vi "Set LV Color.vi"(8 "error in (no error)":errorcluster, 10 "Color (black)":u32(colorbox), 11 "RGB Color.lvclass in":refnum<class "RGB Color.lvclass">) -> (0 "error out":errorcluster, 3 "RGB Color.lvclass out":refnum<class "RGB Color.lvclass">)   [LabVIEW 2018, in "RGB Color.lvclass"]
doc: "A method to set the color from a LabVIEW color value. If the same color cannot be shown in the color model, the closest color will be selected."
uses:
  RGB Color.lvclass
  RGB Color.lvclass/RGB Color.ctl
panel:
  # "expressionflow.com"
  # "Copyright (c) 2008 Tomi Maila. All rights reserved."
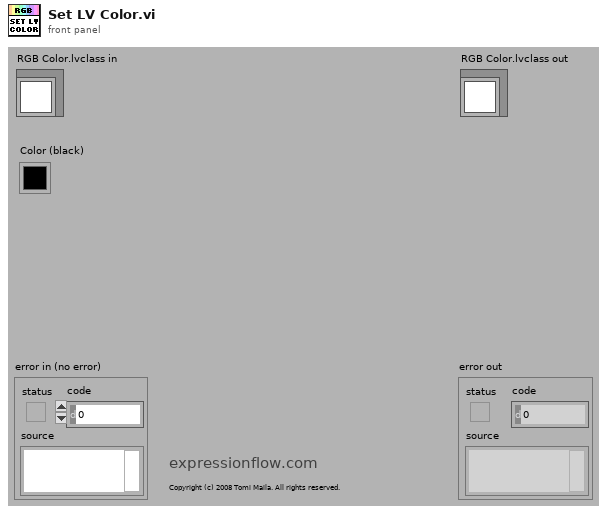
[diagram p1: front panel]
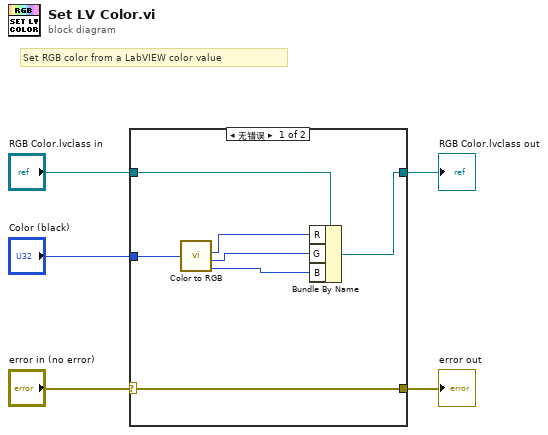
[diagram p0: block diagram]
diagram:
  # "Set RGB color from a LabVIEW color value"
  n1 = case shown="无错误" "error in (no error)" {
    selector: "error in (no error)" -> [w12 w13]
    tunnel: [w12 w13] -> w4
    tunnel: "RGB Color.lvclass in" -> [w11 w14]
    tunnel: [w10 w14] -> w2
    tunnel: "Color (black)" -> [w9 _]
    frame No Error {
      n2 = call <vilib>:"Color to RGB.vi"("Color"=w9) -> ("R"=w8:u8, "G"=w7:u8, "B"=w6:u8)  [unwired: 1 out]
      n3 = Bundle By Name(cluster=w11, "R"=w8, "G"=w7, "B"=w6) -> (w10:refnum<class "RGB Color.lvclass">)
    }
    frame Error {
    }
  }
  "error out" <- w4
  "RGB Color.lvclass out" <- w2
